vi "API Definition.vi"   [LabVIEW 2015, in "LVJSON.lvlib"]
uses:
  LVJSON.lvlib
  JSON Data Classes/JSON Datatype/JSON Datatype.lvclass
  JSON Data Classes/JSON Array/JSON Array.lvclass
  JSON Data Classes/JSON Basic Type/JSON Basic Type.lvclass
  JSON Data Classes/JSON Datatype/To More Specific Type (String).vi
  JSON Data Classes/JSON Datatype/To More Specific Type (Numeric).vi
  JSON Data Classes/JSON Datatype/To More Specific Type (Boolean).vi
  JSON Data Classes/JSON Datatype/To More Specific Type (NULL).vi
  JSON Data Classes/JSON Datatype/To More Specific Type (Array).vi
  JSON Data Classes/JSON Datatype/To More Specific Type (Object).vi
  JSON Data Classes/JSON String/New JSON String.vi
  JSON Data Classes/JSON String/JSON String.lvclass
  JSON Data Classes/JSON Numeric/New JSON Numeric.vi
  JSON Data Classes/JSON Numeric/JSON Numeric.lvclass
  JSON Data Classes/JSON Boolean/New JSON Boolean.vi
  JSON Data Classes/JSON Boolean/JSON Boolean.lvclass
  JSON Data Classes/JSON Null/New JSON Null.vi
  JSON Data Classes/JSON Null/JSON Null.lvclass
  JSON Data Classes/JSON Object/New JSON Object (Empty).vi
  JSON Data Classes/JSON Object/JSON Object.lvclass
  JSON Data Classes/JSON Numeric/Read value (Numeric).vi
  JSON Data Classes/JSON Boolean/Read value (Boolean).vi
  JSON Data Classes/JSON Array/Index Array (Numeric).vi
  JSON Data Classes/JSON Array/Index Array (Boolean).vi
  JSON Data Classes/JSON Array/Index Array (1D Array).vi
  JSON Data Classes/JSON Array/New JSON Array (JSON Data).vi
  JSON Data Classes/JSON Array/New JSON Array (Boolean).vi
  JSON Data Classes/JSON Array/New JSON Array (Numeric).vi
  JSON Data Classes/JSON Array/New JSON Array (String).vi
  JSON Data Classes/JSON Array/New JSON Array (Empty).vi
  JSON Data Classes/JSON Object/New JSON Object (Single).vi
  JSON Data Classes/JSON Object/New JSON Object (Multi).vi
  JSON Data Classes/JSON Array/Index Array (Object).vi
  JSON Data Classes/JSON Array/Insert Into Array (Single).vi
  JSON Data Classes/JSON String/Read value (String).vi
  JSON Data Classes/JSON Array/Build Array (Single).vi
  JSON Data Classes/JSON Object/Insert Key Value Pair (Single).vi
  JSON Data Classes/JSON Object/Get Value (Numeric).vi
  JSON Data Classes/JSON Object/Get Value (Boolean).vi
  JSON Data Classes/JSON Object/Get Value (JSON).vi
  JSON Data Classes/JSON Array/Delete from Array (Single).vi
  JSON Data Classes/JSON Array/Replace Array Subset (Single).vi
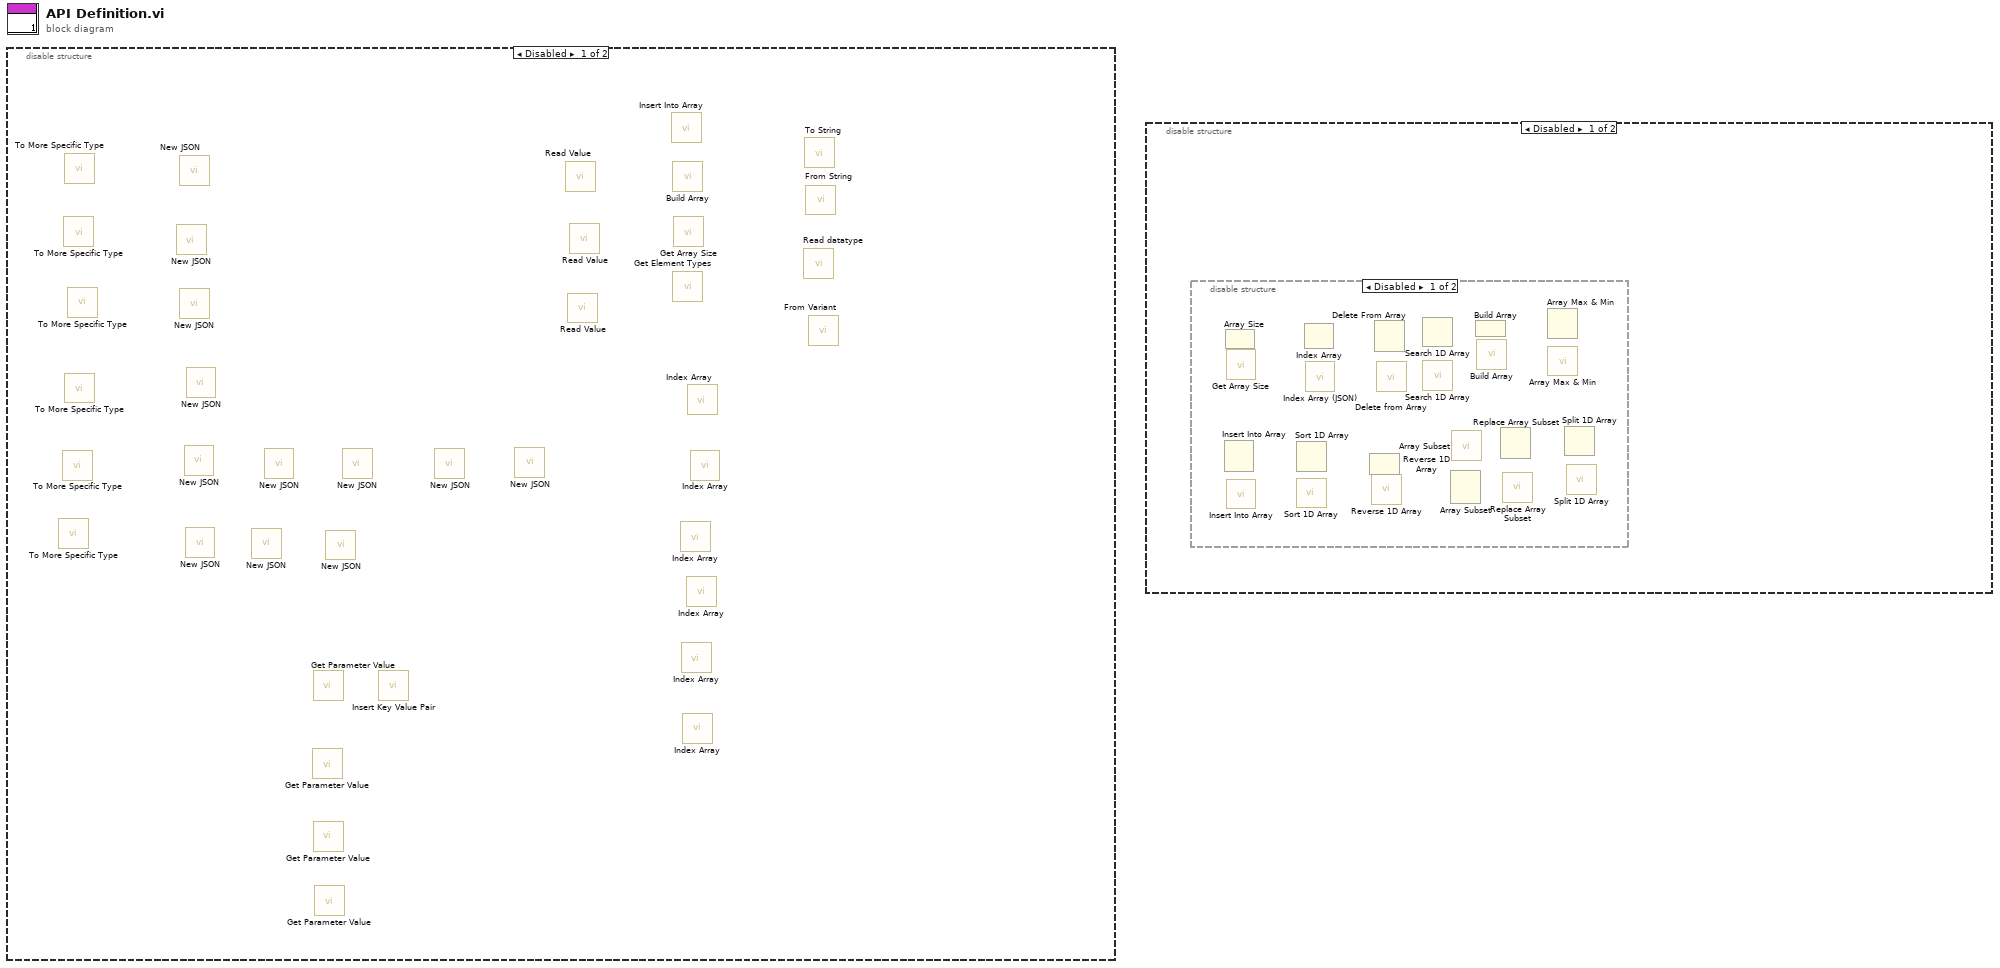
[diagram p0: block diagram]
diagram:
  n1 = disable-structure shown="Disabled" {
    frame Disabled {
      n2 = call-poly "To More Specific Type.vi"() -> ()  [unwired: 10 in, 2 out]
      n3 = call-poly "To More Specific Type.vi"() -> ()  [unwired: 10 in, 2 out]
      n4 = call-poly "To More Specific Type.vi"() -> ()  [unwired: 10 in, 2 out]
      n5 = call-poly "To More Specific Type.vi"() -> ()  [unwired: 10 in, 2 out]
      n6 = call-poly "To More Specific Type.vi"() -> ()  [unwired: 10 in, 2 out]
      n7 = call-poly "To More Specific Type.vi"() -> ()  [unwired: 10 in, 2 out]
      n8 = call-poly "New JSON.vi"() -> ()  [unwired: 10 in, 2 out]
      n9 = call-poly "New JSON.vi"() -> ()  [unwired: 10 in, 2 out]
      n10 = call-poly "New JSON.vi"() -> ()  [unwired: 10 in, 2 out]
      n11 = call-poly "New JSON.vi"() -> ()  [unwired: 10 in, 2 out]
      n12 = call-poly "New JSON.vi"() -> ()  [unwired: 10 in, 2 out]
      n13 = call-poly "New JSON.vi"() -> ()  [unwired: 10 in, 2 out]
      n14 = call-poly "New JSON.vi"() -> ()  [unwired: 10 in, 2 out]
      n15 = call-poly "New JSON.vi"() -> ()  [unwired: 10 in, 2 out]
      n16 = call-poly "Get Parameter Value.vi"() -> ()  [unwired: 9 in, 3 out]
      n17 = call-poly "Get Parameter Value.vi"() -> ()  [unwired: 9 in, 3 out]
      n18 = call-poly "Get Parameter Value.vi"() -> ()  [unwired: 9 in, 3 out]
      n19 = call-poly "Get Parameter Value.vi"() -> ()  [unwired: 9 in, 3 out]
      n20 = call-poly "New JSON.vi"() -> ()  [unwired: 10 in, 2 out]
      n21 = call-poly "New JSON.vi"() -> ()  [unwired: 10 in, 2 out]
      n22 = call-poly "Insert Key Value Pair.vi"() -> ()  [unwired: 10 in, 2 out]
      n23 = call-poly "New JSON.vi"() -> ()  [unwired: 10 in, 2 out]
      n24 = call-poly "New JSON.vi"() -> ()  [unwired: 10 in, 2 out]
      n25 = call-poly "Read Value.vi"() -> ()  [unwired: 9 in, 3 out]
      n26 = call-poly "Read Value.vi"() -> ()  [unwired: 9 in, 3 out]
      n27 = call-poly "Read Value.vi"() -> ()  [unwired: 9 in, 3 out]
      n28 = call-poly "Insert Into Array.vi"() -> ()  [unwired: 11 in, 1 out]
      n29 = call-poly "Build Array.vi"() -> ()  [unwired: 6 in, 1 out]
      n30 = call "Get Element Types.vi"() -> ()  [unwired: 8 in, 4 out]
      n31 = call "Get Array Size.vi"() -> ()  [unwired: 1 in, 1 out]
      n32 = call-poly "Index Array.vi"() -> ()  [unwired: 10 in, 2 out]
      n33 = call-poly "Index Array.vi"() -> ()  [unwired: 10 in, 2 out]
      n34 = call-poly "Index Array.vi"() -> ()  [unwired: 11 in, 1 out]
      n35 = call-poly "Index Array.vi"() -> ()  [unwired: 10 in, 2 out]
      n36 = call-poly "Index Array.vi"() -> ()  [unwired: 11 in, 1 out]
      n37 = call-poly "Index Array.vi"() -> ()  [unwired: 10 in, 2 out]
      n38 = call-dynamic "Read datatype.vi"() -> ()  [unwired: 9 in, 3 out]
      n39 = call-dynamic "To String.vi"() -> ()  [unwired: 10 in, 2 out]
      n40 = call "From String.vi"() -> ()  [unwired: 10 in, 2 out]
      n41 = call "From Variant.vi"() -> ()  [unwired: 10 in, 2 out]
    }
    frame Enabled {
    }
  }
  n42 = disable-structure shown="Disabled" {
    frame Disabled {
      n43 = disable-structure shown="Disabled" {
        frame Disabled {
          n44 = Insert Into Array() -> ()  [unwired: 3 in, 1 out]
          n45 = Array Size() -> ()  [unwired: 1 in, 1 out]
          n46 = call "Get Array Size.vi"() -> ()  [unwired: 1 in, 1 out]
          n47 = call-poly "Insert Into Array.vi"() -> ()  [unwired: 11 in, 1 out]
          n48 = Sort 1D Array() -> ()  [unwired: 1 in, 1 out]
          n49 = call "Sort 1D Array.vi"() -> ()  [unwired: 14 in, 2 out]
          n50 = Index Array() -> ()  [unwired: 2 in, 1 out]
          n51 = call "Index Array (JSON).vi"() -> ()  [unwired: 11 in, 1 out]
          n52 = Reverse 1D Array() -> ()  [unwired: 1 in, 1 out]
          n53 = call "Reverse 1D Array.vi"() -> ()  [unwired: 15 in, 1 out]
          n54 = Delete From Array() -> ()  [unwired: 3 in, 2 out]
          n55 = call-poly "Delete from Array.vi"() -> ()  [unwired: 10 in, 2 out]
          n56 = Search 1D Array() -> ()  [unwired: 3 in, 1 out]
          n57 = call "Search 1D Array.vi"() -> ()  [unwired: 15 in, 1 out]
          n58 = Array Subset() -> ()  [unwired: 3 in, 1 out]
          n59 = call "Array Subset.vi"() -> ()  [unwired: 15 in, 1 out]
          n60 = Build Array() -> ()  [unwired: 2 in, 1 out]
          n61 = call-poly "Build Array.vi"() -> ()  [unwired: 6 in, 1 out]
          n62 = Replace Array Subset() -> ()  [unwired: 3 in, 1 out]
          n63 = call-poly "Replace Array Subset.vi"() -> ()  [unwired: 15 in, 1 out]
          n64 = Array Max & Min() -> ()  [unwired: 1 in, 4 out]
          n65 = call "Array Max & Min.vi"() -> ()  [unwired: 11 in, 5 out]
          n66 = Split 1D Array() -> ()  [unwired: 2 in, 2 out]
          n67 = call "Split 1D Array.vi"() -> ()  [unwired: 14 in, 2 out]
        }
        frame Enabled {
        }
      }
    }
    frame Enabled {
    }
  }
